vi "DEMO-Array Drag.vi"() -> ()   [LabVIEW 2020]
panel:
  in  "stop":bool
  in  "Array":cluster{"Numeric Control":dbl}[](array[cluster])=[{"Numeric Control"=1.0}, {"Numeric Control"=2.0}, {"Numeric Control"=3.0}, {"Numeric Control"=4.0}, {"Numeric Control"=5.0}]
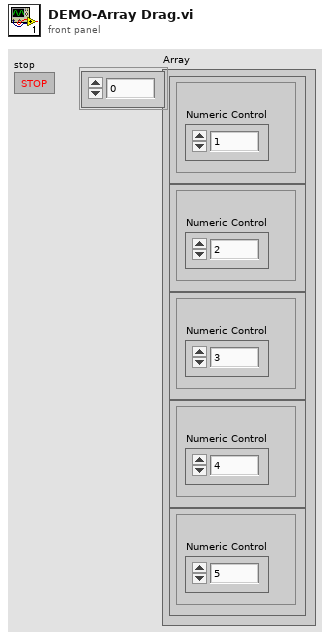
[diagram p1: front panel]
types:
  T1 = typedef "LVPoint32TypeDef.ctl" = cluster{"Horizontal":i32, "Vertical":i32}
  T2 = cluster{"data name":string, "drag data":variant}[]
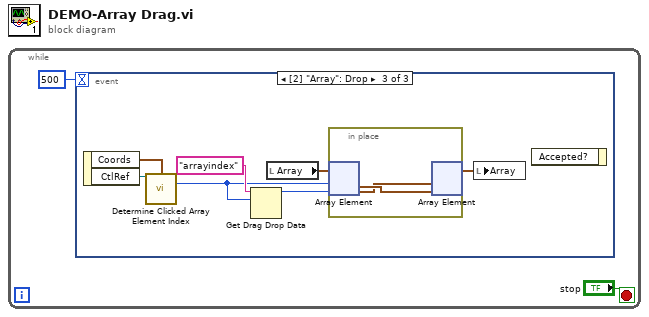
[diagram p0: block diagram]
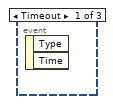
[diagram p2: hidden frame]
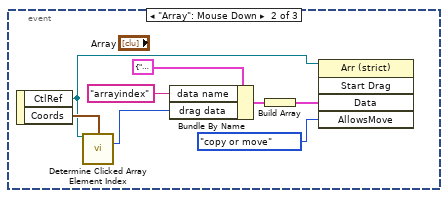
[diagram p3: hidden frame]
diagram:
  n1 = while {
    stop <- "stop" stop-if-true
    n2 = event shown="[2] \"Array\": Drop" {
      selector: _ -> [_ _ _]
      dyn-events: _ -> [_ _ _]
      timeout: 500 -> [_ _ _]
      event Timeout {
        n3 = event-data() -> ()  [unwired: 1 in, 2 out]
      }
      event "Array": Mouse Down {
        n4 = event-data() -> ("CtlRef"=w4:refnum<vi>, "Coords"=w10:T1)  [unwired: 1 in]
        n5 = call "Determine Clicked Array Element Index.vi"("reference"=w4, "Coords of Click"=w10) -> ("Clicked Row"=w5:i32)  [unwired: 8 in, 5 out]
        n6 = Bundle By Name(cluster=cluster{"data name":string, "drag data":variant} {"data name"="", "drag data"=variant}, "data name"="arrayindex", "drag data"=w5) -> (w8:cluster{"data name":string, "drag data":variant})
        n7 = Build Array(w8) -> (w7:T2)
        n8 = invoke on="Invoke Node" class="Arr (strict)" method="Start Drag"(reference=w4, "Data"=w7, "AllowsMove"=enum32{"copy or move", "copy only", "move only"}."copy or move" ("Drag Mode")) -> ()  [unwired: 2 in, 5 out]
      }
      event "Array": Drop {
        n9 = event-data() -> ("Coords"=w11:T1, "CtlRef"=w17:refnum<vi>)  [unwired: 1 in]
        n10 = call "Determine Clicked Array Element Index.vi"("reference"=w17, "Coords of Click"=w11) -> ("Clicked Row"=w12:i32)  [unwired: 8 in, 5 out]
        n11 = Get Drag Drop Data(8:w12, 9:"arrayindex" ("data name")) -> (3:w14:i32)  [unwired: 1 in, 1 out]
        n12 = local read "Array"() -> (w15:cluster{"Numeric Control":dbl}[])
        n13 = in-place {
          n14 = in-place-array #1(w15, w12, w14) -> (w19:cluster{"Numeric Control":dbl}, w18:cluster{"Numeric Control":dbl})
          n15 = in-place-array #1(w18, w19) -> (w16:cluster{"Numeric Control":dbl}[])  [unwired: 2 out]
        }
        n16 = local write "Array"(w16) -> ()
        n17 = event-data() -> ()  [unwired: 2 in, 1 out]
      }
    }
  }
